vi "Saturation_Count.vi"() -> ()   [LabVIEW 2014]
panel:
  out "Saturation Count":dbl
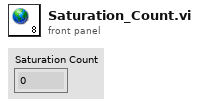
[diagram p1: front panel]
diagram:
